vi "Get VI In and Outputs.vi"(8 "error in (no error)":errorcluster, 11 "VI in":refnum<vi>) -> (0 "error out":errorcluster, 2 "Controls":refnum<vi>[](array[refnum]), 3 "Indicators":refnum<vi>[](array[refnum]))   [LabVIEW 2025, in "Scripting Server.lvlib" / "Tools.lvlib"]
uses:
  Tools.lvlib
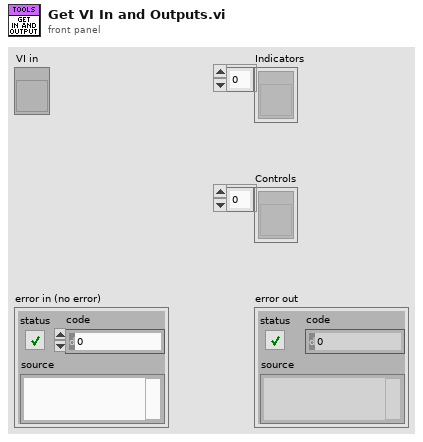
[diagram p1: front panel]
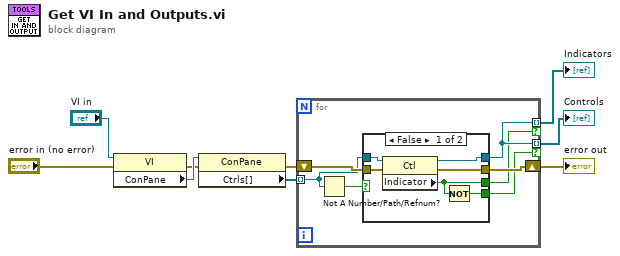
[diagram p0: block diagram]
diagram:
  n1 = property class="VI"(reference="VI in", error in="error in (no error)") -> (error out=w7:errorcluster, "ConPane"=w9:refnum<vi>)  [unwired: 1 out]
  n2 = property class="ConPane"(reference=w9, error in=w7) -> (error out=w2:errorcluster, "Ctrls[]"=w3:refnum<vi>[])  [unwired: 1 out]
  n3 = for {
    shift-right: [w15] -> w5
    shift-left: w2 -> [w16]
    tunnel: w3 -> [w11] mode=indexing
    tunnel: [w14] -> w4 mode=indexing if=w13
    tunnel: [w14] -> w6 mode=indexing if=w12
    n4 = Not A Number/Path/Refnum?(number/path/refnum=w11) -> (NaN/Path/Refnum?=w10:bool)
    n5 = case shown="False" w10 {
      tunnel: w16 -> [w22 w23]
      tunnel: [w21 w23] -> w15
      tunnel: w11 -> [w20 _]
      tunnel: [w19 _] -> w14
      tunnel: [w18 _] -> w13
      tunnel: [w17 _] -> w12
      frame False {
        n6 = property class="Ctl"(reference=w20, error in=w22) -> (reference out=w19:refnum<vi>, error out=w21:errorcluster, "Indicator"=w18:bool)
        n7 = Not(x=w18) -> (.not. x?=w17:bool)
      }
      frame True {
      }
    }
  }
  "Controls" <- w6
  "error out" <- w5
  "Indicators" <- w4
